vi "SC10_get_state2.vi"() -> ()   [LabVIEW 2010]
panel:
  out "state (numeric)":i32
  out "state":string
  in  "VISA resource name":refnum<visa-resource-name>
  out "VISA resource name out":refnum<visa-resource-name>
  out "read buffer":string
  out "return count 2":u32
  out "return count":u32
  out "error out":errorcluster
  in  "error in (no error)":errorcluster
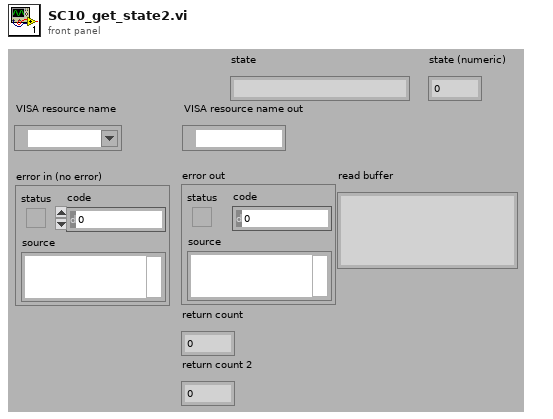
[diagram p1: front panel]
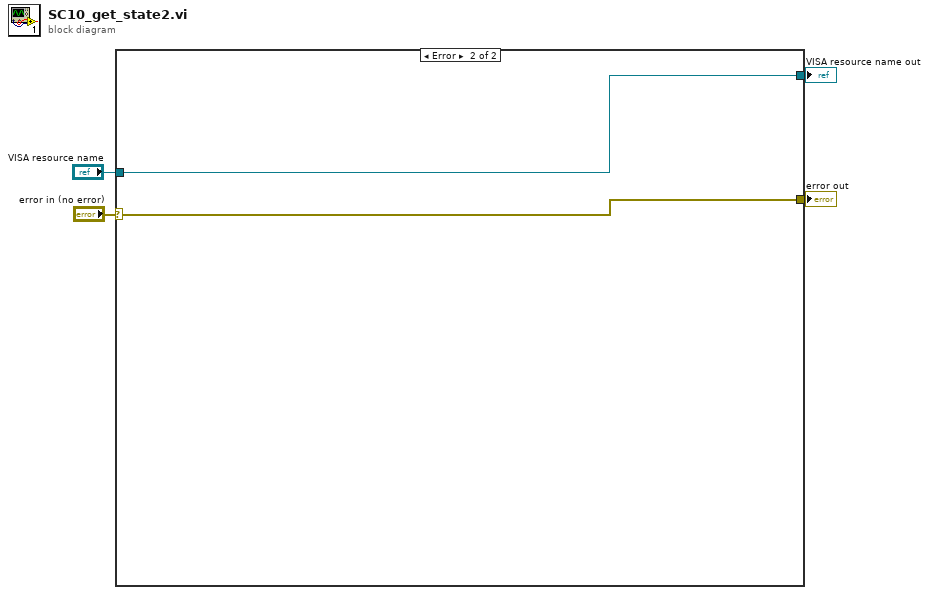
[diagram p0: block diagram]
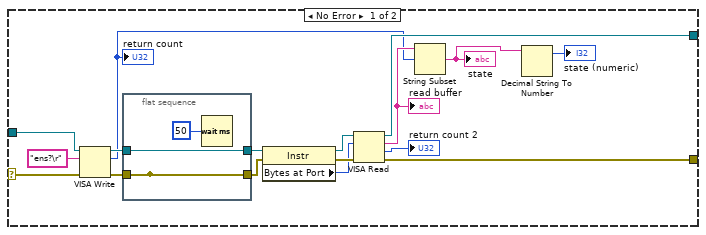
[diagram p2: hidden frame]
diagram:
  n1 = case shown="Error" "error in (no error)" {
    selector: "error in (no error)" -> [w19 w25]
    tunnel: [w18 w25] -> w3
    tunnel: [w16 w26] -> w2
    tunnel: "VISA resource name" -> [w15 w26]
    frame No Error {
      n2 = VISA Write(VISA resource name=w15, write buffer="ens?\r", error in (no error)=w19) -> (VISA resource name out=w21:refnum<visa-resource-name>, return count=w13:u32, error out=w20:errorcluster)
      "return count" <- w13
      n3 = flat-sequence {
        tunnel: w21 -> [w23]
        tunnel: [w23] -> w10
        tunnel: w20 -> [w22]
        tunnel: [w22] -> _
        tunnel: [w22] -> w7
        frame #0 {
          n4 = Wait (ms)(milliseconds to wait=u32 50) -> ()  [unwired: 1 out]
        }
      }
      n5 = property class="Instr"(reference=w10, error in=w7) -> (reference out=w11:refnum<visa-resource-name>, error out=w9:errorcluster, "Bytes at Port"=w8:u32)
      n6 = VISA Read(VISA resource name=w11, byte count=w8, error in (no error)=w9) -> (VISA resource name out=w16:refnum<visa-resource-name>, read buffer=w14:string, return count=→"return count 2":u32, error out=w18:errorcluster)
      "read buffer" <- w14
      n7 = String Subset(string=w14, offset (0)=w13) -> (substring=w6:string)  [unwired: 1 in]
      "state" <- w6
      n8 = Decimal String To Number(string=w6) -> (offset past number=→"state (numeric)":i32)  [unwired: 2 in, 1 out]
    }
    frame Error {
    }
  }
  "error out" <- w3
  "VISA resource name out" <- w2
